vi "preconditioning_practice.vi"() -> ()   [LabVIEW 2014]
uses:
  <vilib>/Motion/FlexMotion/CustomControls/CustomControls.llb/AxisOrVectorSpace To Configure.flx
  <vilib>/Motion/FlexMotion/FunctionsVIs/StartStopMotion.llb/Start Motion (8 axes).flx
  <vilib>/Motion/FlexMotion/FunctionsVIs/Trajectory.llb/Check Move Complete Status (8 axes).flx
  <vilib>/Motion/FlexMotion/FunctionsVIs/StartStopMotion.llb/Stop Motion (8 axes).flx
panel:
  out "estimated time per step":dbl
  in  "Velocity mm/s":dbl
  in  "Displacement":dbl
  in  "Number of cycles":i32
  out "millisecond timer value":u32
  in  "Number of steps in each cycle":i32
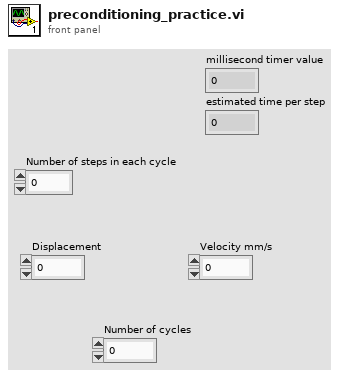
[diagram p1: front panel]
types:
  T1 = typedef "AxisOrVectorSpace To Configure.flx" = u16
  T2 = typedef "Board Id" = u8
  T3 = enum16{"Absolute Position", "Relative Position", "Velocity", "Relative to Cap Pos", "Modulus Position", "Absolute Contouring", "Relative Contouring"}
  T4 = typedef "Resource Out (Enum).flx" = u16
  T5 = typedef "Bd Id Out" = u8
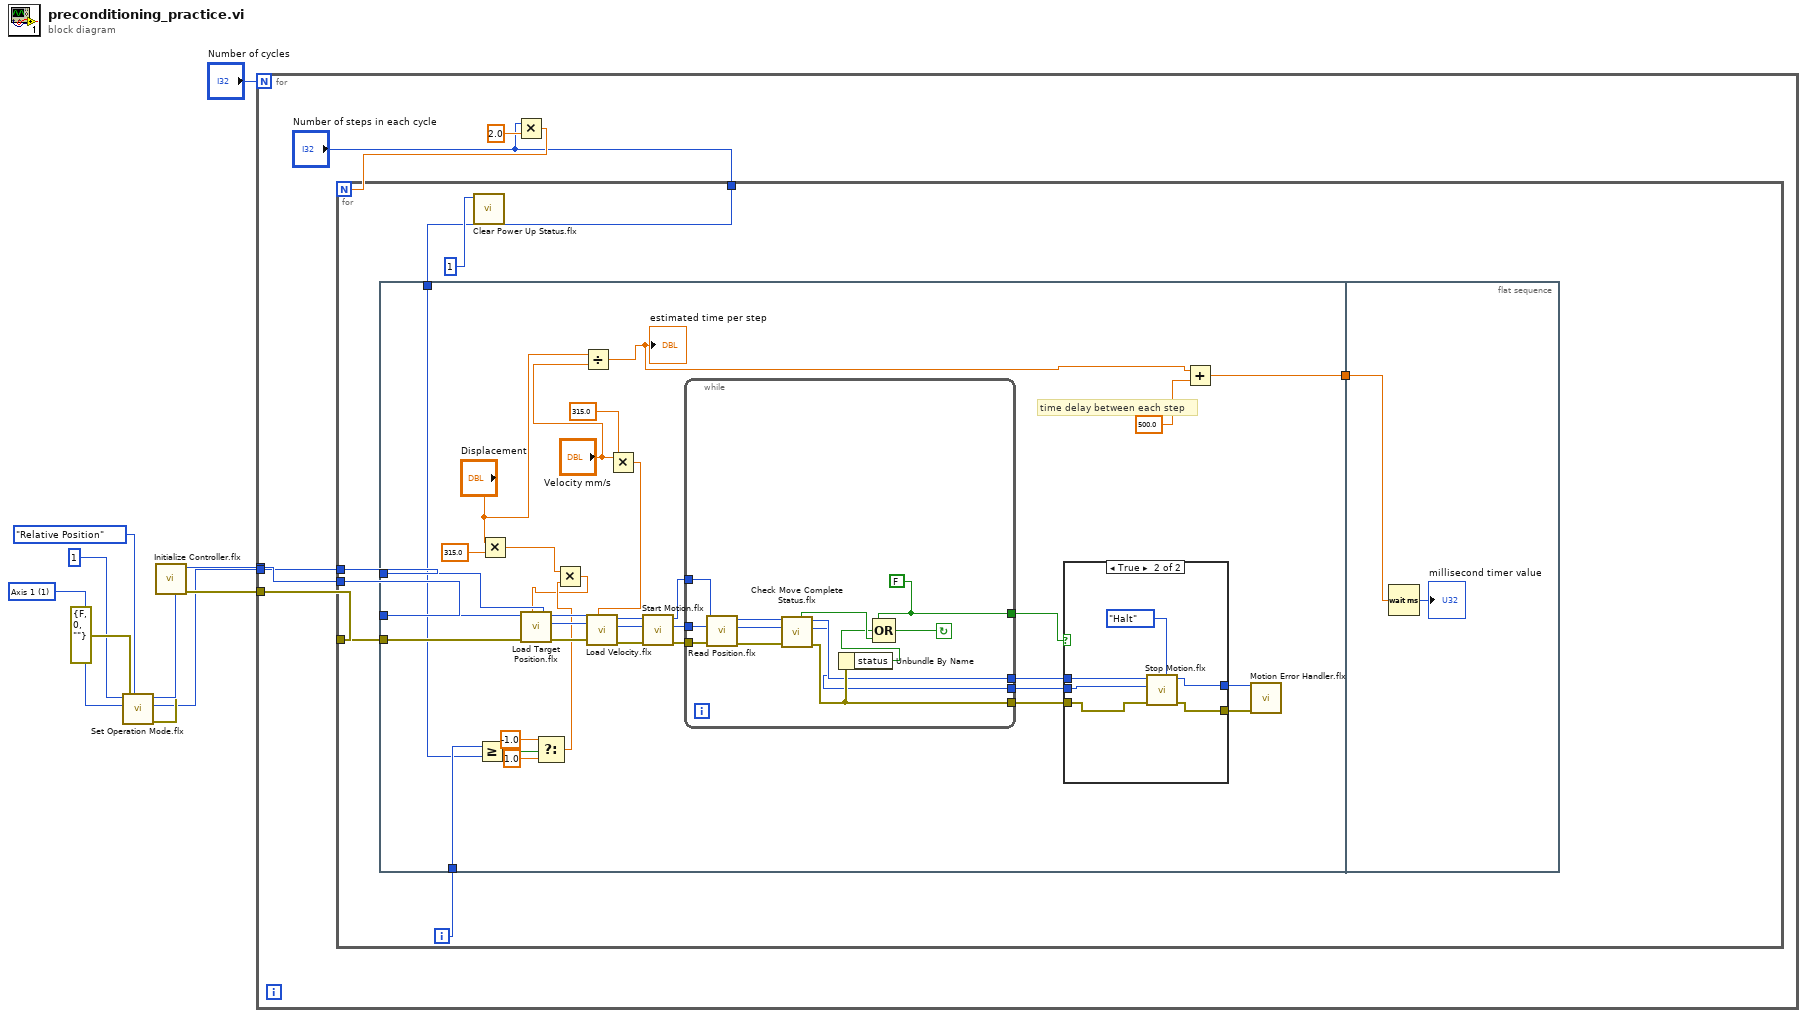
[diagram p0: block diagram]
diagram:
  w7 = T1 1 items=["Axis 1"=1, "Axis 2"=2, "Axis 3"=3, "Axis 4"=4, "Axis 5"=5, "Axis 6"=6, "Axis 7"=7, "Axis 8"=8, "Vector Space 1"=17, "Vector Space 2"=18, "Vector Space 3"=19, "Vector Space 4"=20] ("Axis or Vector Space")
  n1 = call <vilib>:"Set Operation Mode.flx"("Position Mode (Absolute)"=T3."Relative Position", "error in (no error)"=errorcluster {"status"=FALSE, "code"=0, "source"=""} ("error constant"), "Axis or Vector Space"=w7, "Board ID"=T2 1) -> ("error out"=w9:errorcluster, "Resource Output"=w2:T4, "Bd ID Out"=w10:T5)  [unwired: 2 in]
  n2 = call <vilib>:"Initialize Controller.flx"("error in (no error)"=w9, "Board ID"=w10) -> ("error out"=w3:errorcluster, "Bd ID Out"=w4:T5)  [unwired: 6 in]
  n3 = for {
    N: "Number of cycles" -> [_]
    tunnel: w4 -> [w16]
    tunnel: w3 -> [w15]
    tunnel: w2 -> [w14]
    n4 = Multiply(x="Number of steps in each cycle", y=2.0) -> (x*y=w12:dbl)
    n5 = for {
      N: w12 -> [_]
      tunnel: w16 -> [w22]
      tunnel: w15 -> [w21]
      tunnel: w14 -> [w20]
      tunnel: "Number of steps in each cycle" -> [w18]
      i -> [w19]
      n6 = flat-sequence {
        tunnel: w19 -> [w39]
        tunnel: w18 -> [w38]
        tunnel: w22 -> [w42]
        tunnel: w21 -> [w41]
        tunnel: w20 -> [w40]
        tunnel: [w24] -> w17
        tunnel: w17 -> [w79]
        frame #0 {
          # "time delay between each step"
          n7 = Greater Or Equal?(x=w39, y=w38) -> (x >= y?=w37:bool)
          n8 = Multiply(x="Displacement", y=315.0) -> (x*y=w31:dbl)
          n9 = Select(t=-1.0, s=w37, f=1.0) -> (s? t:f=w34:dbl)
          n10 = Multiply(x=w31, y=w34) -> (x*y=w33:dbl)
          n11 = call <vilib>:"Load Target Position.flx"("Target Position (0)"=w33, "error in (no error)"=w41, "Axis"=w40, "Board ID"=w42) -> ("error out"=w55:errorcluster, "Resource Output"=w56:T4, "Bd ID Out"=w57:T5)  [unwired: 3 in]
          n12 = Divide(x="Displacement", y="Velocity mm/s") -> (x/y=w25:dbl)
          "estimated time per step" <- w25
          n13 = Multiply(x="Velocity mm/s", y=315.0) -> (x*y=w28:dbl)
          n14 = call <vilib>:"Load Velocity.flx"("Velocity (10000)"=w28, "error in (no error)"=w55, "Axis or Vector Space"=w56, "Board ID"=w57) -> ("error out"=w52:errorcluster, "Resource Output"=w53:T4, "Bd ID Out"=w54:T5)  [unwired: 3 in]
          n15 = call-poly <vilib>:"Start Motion.flx"("error in (no error)"=w52, "Axis or Vector Space"=w53, "Board ID"=w54) -> ("error out"=w49:errorcluster, "Resource Output"=w50:T4, "Bd ID Out"=w51:T5)  [unwired: 3 in]
          n16 = while {
            tunnel: w51 -> [w78]
            tunnel: w50 -> [w77]
            tunnel: w49 -> [w76]
            tunnel: [w70] -> w48
            tunnel: [w69] -> w47
            tunnel: [w67] -> w46
            tunnel: [w66] -> w45
            stop <- w71 continue-if-true
            w70 = FALSE
            n17 = call <vilib>:"Read Position.flx"("error in (no error)"=w76, "Axis"=w77, "Board ID"=w78) -> ("error out"=w73:errorcluster, "Resource Output"=w74:T4, "Bd ID Out"=w75:T5)  [unwired: 3 in, 1 out]
            n18 = call-poly <vilib>:"Check Move Complete Status.flx"("error in (no error)"=w73, "Axis or Vector Space"=w74, "Board ID"=w75) -> ("error out"=w69:errorcluster, "Resource Output"=w66:T4, "Bd ID Out"=w67:T5, "Move Complete"=w72:bool)  [unwired: 3 in]
            n19 = Unbundle By Name(w69) -> ("status"=w68:bool)
            n20 = Compound Arithmetic op=OR(w70, w68, w72) -> (w71:bool)
          }
          n21 = case shown="True" w48 {
            tunnel: w47 -> [w58 w65]
            tunnel: w46 -> [w59 w64]
            tunnel: w45 -> [_ w63]
            tunnel: [w58 w62] -> w44
            tunnel: [w59 w61] -> w43
            frame False {
            }
            frame True {
              n22 = call-poly <vilib>:"Stop Motion.flx"("Stop Type (Decel)"=enum16{"Decelerate", "Halt", "Kill"}."Halt", "error in (no error)"=w65, "Axis or Vector Space"=w63, "Board ID"=w64) -> ("error out"=w62:errorcluster, "Bd ID Out"=w61:T5)  [unwired: 3 in, 1 out]
            }
          }
          n23 = Add(x=w25, y=500.0) -> (x+y=w24:dbl)
          n24 = call <vilib>:"Motion Error Handler.flx"("Board ID"=w43, "error in (no error)"=w44) -> ()  [unwired: 9 in, 5 out]
        }
        frame #1 {
          n25 = Wait (ms)(milliseconds to wait=w79) -> (millisecond timer value=→"millisecond timer value":u32)
        }
      }
      n26 = call <vilib>:"Clear Power Up Status.flx"("Board ID"=T2 1) -> ()  [unwired: 6 in, 2 out]
    }
  }
